vi "Control_Xbox.vi"() -> ()   [LabVIEW 2016]
uses:
  <vilib>/Utility/inputDevices.llb/joystickAcquire.vi
  <vilib>/Utility/inputDevices.llb/closeJoystick.vi
panel:
  out "Indice":i32
  in  "Stop Button":bool
  out "direction info":T1
  out "button info":T2
  out "axis info":T3
  out "joystick info":T4(array[cluster])
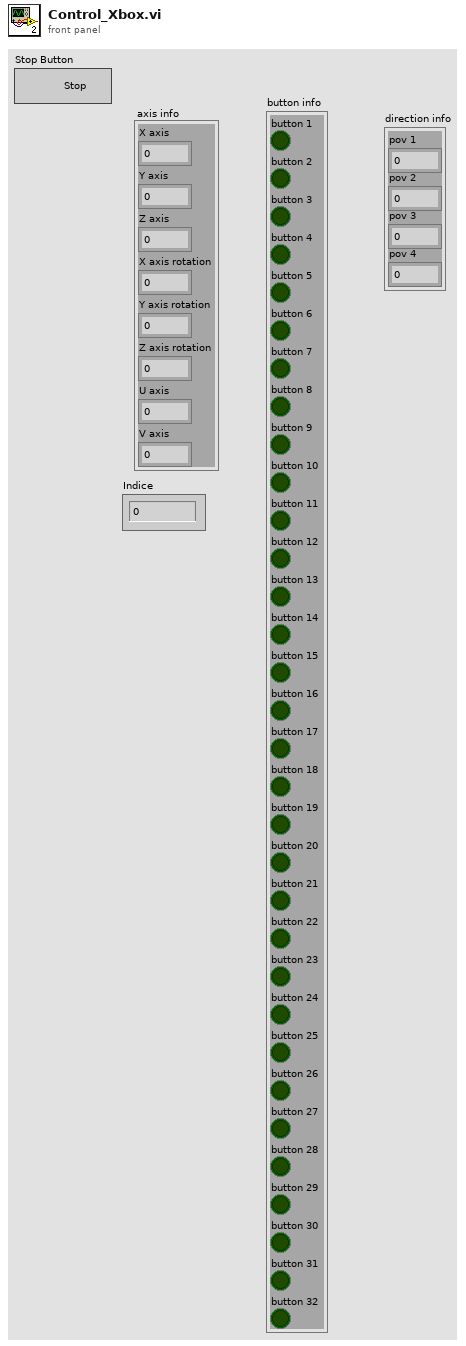
[diagram p1: front panel]
types:
  T1 = cluster{"pov 1":i32, "pov 2":i32, "pov 3":i32, "pov 4":i32}
  T2 = cluster{"button 1":bool, "button 2":bool, "button 3":bool, "button 4":bool, "button 5":bool, "button 6":bool, "button 7":bool, "button 8":bool, "button 9":bool, "button 10":bool, "button 11":bool, "button 12":bool, "button 13":bool, "button 14":bool, "button 15":bool, "button 16":bool, "button 17":bool, "button 18":bool, "button 19":bool, "button 20":bool, "button 21":bool, "button 22":bool, "button 23":bool, "button 24":bool, "button 25":bool, "button 26":bool, "button 27":bool, "button 28":bool, "button 29":bool, "button 30":bool, "button 31":bool, "button 32":bool}
  T3 = cluster{"X axis":i32, "Y axis":i32, "Z axis":i32, "X axis rotation":i32, "Y axis rotation":i32, "Z axis rotation":i32, "U axis":i32, "V axis":i32}
  T4 = cluster{"axes total":u32, "buttons total":u32, "pov total":u32, "device name":string}[]
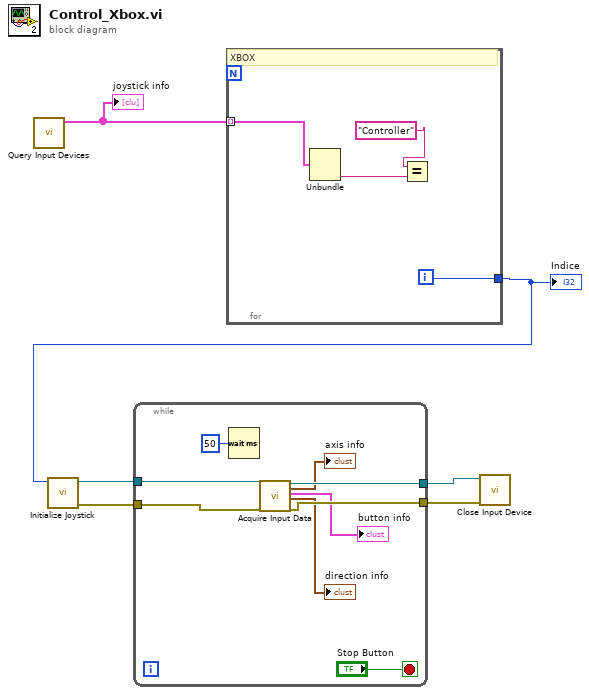
[diagram p0: block diagram]
diagram:
  n1 = call <vilib>:"Query Input Devices.vi"() -> ("joystick info"=w2:T4)  [unwired: 8 in, 3 out]
  "joystick info" <- w2
  n2 = for {
    tunnel: w2 -> [w10] mode=indexing
    tunnel: [w7] -> w1
    i -> [w7]
    # "XBOX"
    n3 = Unbundle(w10) -> ("device name"=w9:string)  [unwired: 3 out]
    n4 = Equal?(x="Controller", y=w9) -> ()  [unwired: 1 out]
  }
  "Indice" <- w1
  n5 = call <vilib>:"Initialize Joystick.vi"("device index"=w1) -> ("error out"=w5:errorcluster, "device ID"=w6:refnum<k1>)  [unwired: 9 in]
  n6 = while {
    tunnel: w6 -> [w19]
    tunnel: w5 -> [w18]
    tunnel: [w17] -> w4
    tunnel: [w16] -> w3
    stop <- "Stop Button" stop-if-true
    n7 = Wait (ms)(milliseconds to wait=u32 50) -> ()  [unwired: 1 out]
    n8 = call-poly <vilib>:"Acquire Input Data.vi"("device ID"=w19, "error in (no error)"=w18) -> ("device ID"=w17:refnum<k1>, "axis info"=→"axis info":T3, "button info"=→"button info":T2, "direction info"=→"direction info":T1, "error out"=w16:errorcluster)  [unwired: 13 in]
  }
  n9 = call-poly <vilib>:"Close Input Device.vi"("error in (no error)"=w3, "device ID"=w4) -> ()  [unwired: 8 in, 1 out]
